vi "wareform de lectura01.vi"() -> ()   [LabVIEW 2020]
panel:
  in  "stop":bool
  out "limite":dbl
  out "alarm":bool
  out "grafica":dynamicdata(graph)
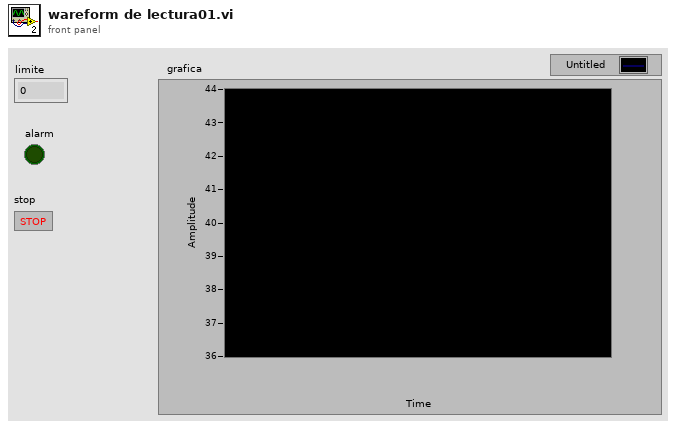
[diagram p1: front panel]
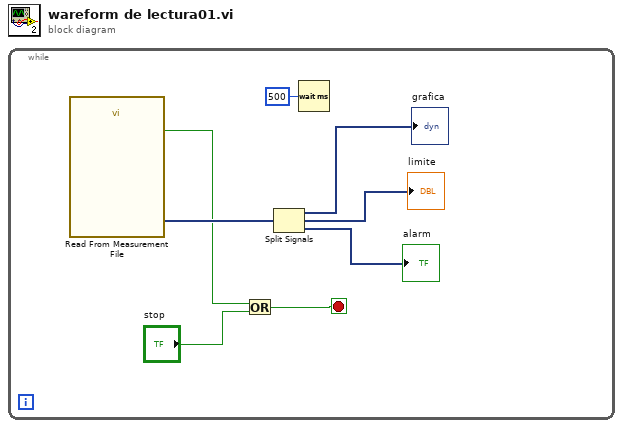
[diagram p0: block diagram]
diagram:
  n1 = while {
    stop <- w3 stop-if-true
    n2 = call "Read From Measurement File"() -> ("Signals"=w7:dynamicdata, "EOF?"=w2:bool)  [unwired: 6 in, 4 out]
    n3 = Or(x=w2, y="stop") -> (x .or. y?=w3:bool)
    n4 = Split Signals(w7) -> (→"grafica":dynamicdata, →"limite":dynamicdata, →"alarm":dynamicdata)  [unwired: 3 in]
    n5 = Wait (ms)(milliseconds to wait=u32 500) -> ()  [unwired: 1 out]
  }
